vi "subPanel - UI Fires Event.vi"(6 "Val(Sgnl)":bool, 8 "Error In":errorcluster, 10 "Pnl Controls[]":refnum<vi>[](array[refnum]), 11 "CtlRef":refnum<vi>) -> (0 "Error Out":errorcluster, 2 "Pnl Controls[]":refnum<vi>[](array[refnum]), 3 "CtlRef":refnum<vi>)   [LabVIEW 2013]
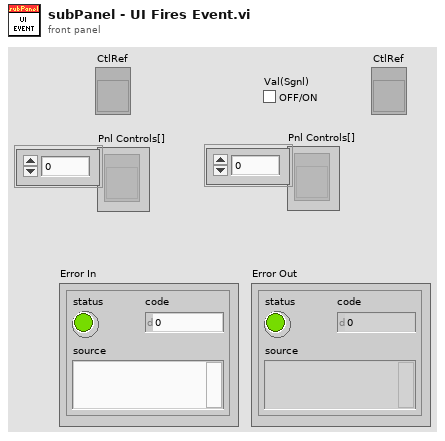
[diagram p1: front panel]
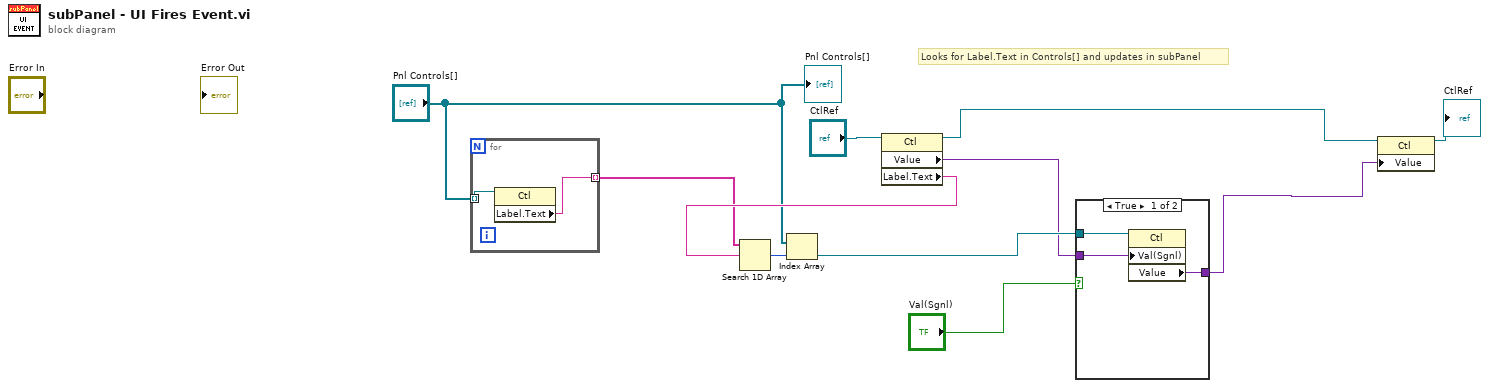
[diagram p0: block diagram]
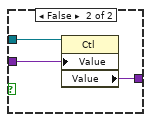
[diagram p2: hidden frame]
diagram:
  # "Looks for Label.Text in Controls[] and updates in subPanel"
  n1 = for {
    tunnel: "Pnl Controls[]" -> [w13] mode=indexing
    tunnel: [w12] -> w3 mode=indexing
    n2 = property class="Ctl"(reference=w13) -> ("Label.Text"=w12:string)  [unwired: 1 in, 2 out]
  }
  n3 = property class="Ctl"(reference="CtlRef") -> (reference out=w7:refnum<vi>, "Value"=w8:variant, "Label.Text"=w5:string)  [unwired: 1 in, 1 out]
  n4 = Search 1D Array(1D array=w3, element=w5) -> (index of element=w10:i32)  [unwired: 1 in]
  n5 = Index Array(array="Pnl Controls[]", index=w10) -> (element=w11:refnum<vi>)
  n6 = case shown="True" "Val(Sgnl)" {
    tunnel: w11 -> [w16 w19]
    tunnel: w8 -> [w15 w18]
    tunnel: [w14 w17] -> w6
    frame True {
      n7 = property class="Ctl"(reference=w16, "Val(Sgnl)"=w15) -> ("Value"=w14:variant)  [unwired: 1 in, 2 out]
    }
    frame False {
      n8 = property class="Ctl"(reference=w19, "Value"=w18) -> ("Value"=w17:variant)  [unwired: 1 in, 2 out]
    }
  }
  n9 = property class="Ctl"(reference=w7, "Value"=w6) -> (reference out=→"CtlRef":refnum<vi>)  [unwired: 1 in, 1 out]
  "Pnl Controls[]" <- "Pnl Controls[]"
